vi "APD_deadtime.vi"(4 "error in":errorcluster) -> (0 "error out":errorcluster, 3 "filtered APD":refnum<k21>)   [LabVIEW 2018]
uses:
  GLOBAL_VAR.vi
  <vilib>/DAQmx/create/channels.llb/DAQmx Create Channel (CO-Pulse Generation-Ticks).vi
  <vilib>/DAQmx/configure/trigger.llb/DAQmx Start Trigger (Digital Edge).vi
  <resource>/objmgr/daqmx.rc
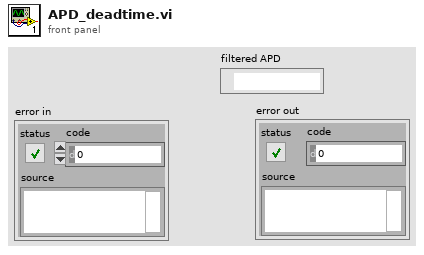
[diagram p1: front panel]
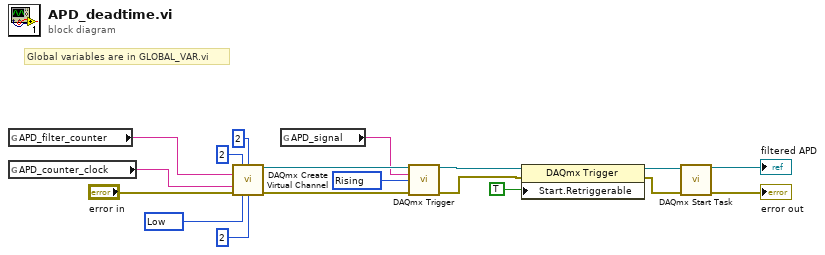
[diagram p0: block diagram]
diagram:
  w8 = 10280 items=["Rising"=10280, "Falling"=10171] ("edge")
  w6 = 10214 items=["High"=10192, "Low"=10214] ("idle state")
  # "Global variables are in GLOBAL_VAR.vi"
  n1 = global read "GLOBAL_VAR.vi" "APD_filter_counter"() -> (w2:tag)
  n2 = global read "GLOBAL_VAR.vi" "APD_counter_clock"() -> (w1:tag)
  n3 = call-poly <vilib>:"DAQmx Create Virtual Channel.vi"("high ticks"=u32 2, "low ticks"=u32 2, "counter"=w2, "source of ticks"=w1, "error in"="error in", "idle state"=w6, "initial delay"=u32 2) -> ("task out"=w12:refnum<k21>, "error out"=w15:errorcluster)  [unwired: 7 in]
  n4 = global read "GLOBAL_VAR.vi" "APD_signal"() -> (w3:tag)
  n5 = call-poly <vilib>:"DAQmx Trigger.vi"("task/channels in"=w12, "source"=w3, "edge"=w8, "error in"=w15) -> ("task out"=w10:refnum<k21>, "error out"=w16:errorcluster)  [unwired: 10 in]
  n6 = property class="DAQmx Trigger"(reference=w10, error in=w16, "Start.Retriggerable"=TRUE) -> (reference out=w13:refnum<k21>, error out=w17:errorcluster)
  n7 = call <vilib>:"DAQmx Start Task.vi"("task/channels in"=w13, "error in"=w17) -> ("task out"=→"filtered APD":refnum<k21>, "error out"=→"error out":errorcluster)  [unwired: 12 in]
